vi "writeToXML.vi"(8 "error in (no error)":errorcluster, 10 "ClassLabel":string, 11 "MccTrack in":refnum<class "MccTrack.lvclass">) -> (0 "error out":errorcluster, 2 "XMLout":string, 3 "MccTrack out":refnum<class "MccTrack.lvclass">)   [LabVIEW 2022 SP3, in "TCSDataDefinitions.lvlib" / "TCSMountControlCommand.lvlib" / "CommandsForAllAxes.lvlib" / "MccTrack.lvclass"]
uses:
  MccTrack.lvclass
  MccTrack.lvclass/MccTrack.ctl
  CommandsForAllAxes.lvclass
  <userlib>/Common/XML/XMLGenerator/XMLGenerator.lvclass
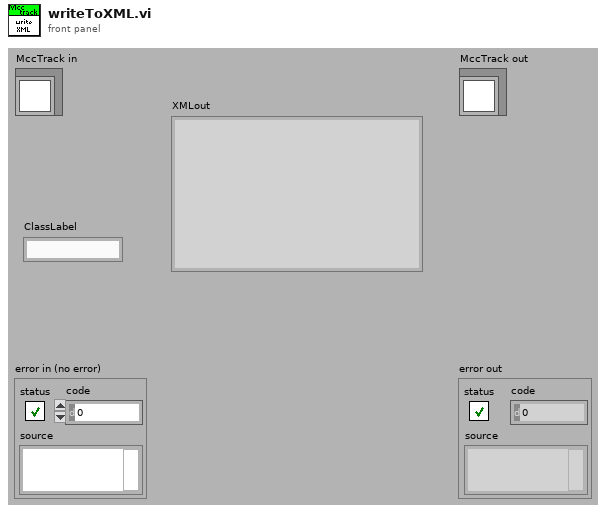
[diagram p1: front panel]
types:
  T1 = typedef "TCSDataDefinitions.lvlib/TCSMountControlCommand.lvlib/MountTrackStates.ctl" = enum16{"On", "Off"}
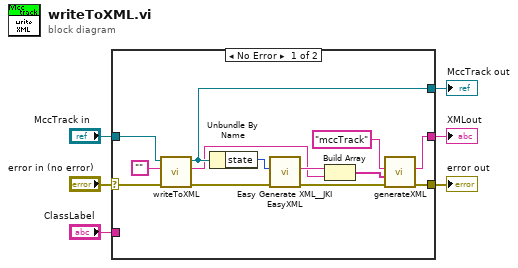
[diagram p0: block diagram]
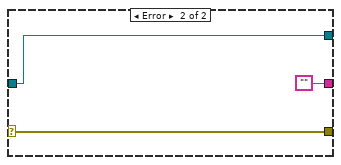
[diagram p2: hidden frame]
diagram:
  n1 = case shown="No Error" "error in (no error)" {
    selector: "error in (no error)" -> [w10 w22]
    tunnel: [w9 w22] -> w5
    tunnel: [w18 w21] -> w3
    tunnel: "MccTrack in" -> [w19 w21]
    tunnel: [w8 ""] -> w2
    tunnel: "ClassLabel" -> [_ _]
    frame No Error {
      n2 = call-parent "writeToXML.vi"("error in (no error)"=w10, "ClassLabel"="", "CommandsForAllAxes in"=w19) -> ("error out"=w16:errorcluster, "XMLout"=w12:string, "CommandsForAllAxes out"=w18:refnum<class "MccTrack.lvclass">)  [unwired: 6 in]
      n3 = Unbundle By Name(w18) -> ("state"=w17:T1)
      n4 = call <vilib>:"Easy Generate XML__JKI EasyXML.vi"("error in (no error)"=w16, "LabVIEW Data"=w17) -> ("error out"=w15:errorcluster, "XML String"=w13:string)  [unwired: 8 in]
      n5 = Build Array(w13, w12) -> (w14:string[])
      n6 = call <userlib>:"generateXML.vi"("error in"=w15, "childrenXML"=w14, "elementName"="mccTrack" ("Class Label")) -> ("error out"=w9:errorcluster, "XML out"=w8:string)  [unwired: 6 in, 1 out]
    }
    frame Error {
    }
  }
  "error out" <- w5
  "MccTrack out" <- w3
  "XMLout" <- w2
